vi "replaceGoto.vi"(10 "String in":string) -> (2 "BotSpeak Out":string)   [LabVIEW 2012]
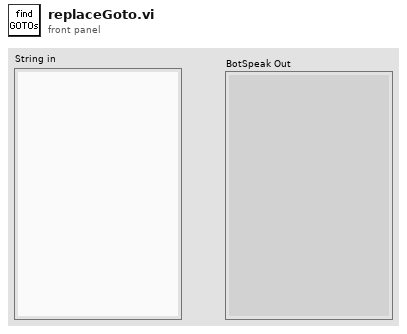
[diagram p1: front panel]
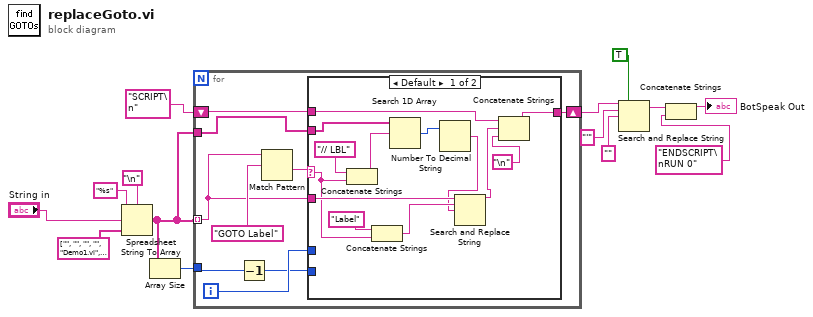
[diagram p0: block diagram]
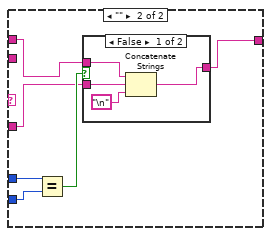
[diagram p2: hidden frame]
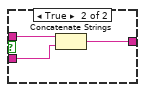
[diagram p3: hidden frame]
diagram:
  n1 = Spreadsheet String To Array(delimiter (Tab)="\n", format string="%s", spreadsheet string="String in", array type (2D Dbl)=string[] ["", "", "", "", "Demo1.vi", "DigitalWrite.vi", "VS_Wait.vi", ""] ("Array 3")) -> (array=w7:string[])
  n2 = Array Size(array=w7) -> (size(s)=w6:i32)
  n3 = for {
    tunnel: w7 -> [w20] mode=indexing
    tunnel: w7 -> [w23]
    shift-right: [w15] -> w2
    shift-left: "SCRIPT\n" -> [w22]
    tunnel: w6 -> [w16]
    i -> [w18]
    n4 = Decrement(x=w16) -> (x-1=w17:i32)
    n5 = Match Pattern(string=w20, regular expression="GOTO Label" ("search string/char (-)")) -> (after substring=w19:string)  [unwired: 1 in, 3 out]
    n6 = case shown="Default" w19 {
      selector: w19 -> [w32 _]
      tunnel: w23 -> [w36 _]
      tunnel: w20 -> [w33 w38]
      tunnel: [w25 w37] -> w15
      tunnel: w22 -> [w27 w39]
      tunnel: w18 -> [_ w42]
      tunnel: w17 -> [_ w41]
      frame Default {
        n7 = Concatenate Strings("// LBL" ("string"), w32) -> (w34:string)
        n8 = Concatenate Strings("Label" ("string"), w32) -> (w30:string)
        n9 = Search 1D Array(1D array=w36, element=w34) -> (index of element=w29:i32)  [unwired: 1 in]
        n10 = Number To Decimal String(number=w29) -> (decimal integer string=w28:string)  [unwired: 1 in]
        n11 = Search and Replace String(input string=w33, search string=w30, replace string=w28) -> (result string=w26:string)  [unwired: 5 in, 3 out]
        n12 = Concatenate Strings(w27, w26, "\n") -> (w25:string)
      }
      frame "" {
        n13 = Equal?(x=w42, y=w41) -> (x = y?=w40:bool)
        n14 = case shown="False" w40 {
          tunnel: w39 -> [w46 w49]
          tunnel: w38 -> [w45 w48]
          tunnel: [w43 w47] -> w37
          frame False {
            n15 = Concatenate Strings(w46, w45, "\n") -> (w43:string)
          }
          frame True {
            n16 = Concatenate Strings(w49, w48) -> (w47:string)
          }
        }
      }
    }
  }
  n17 = Search and Replace String(replace all?=TRUE ("replace all? (F)"), input string=w2, search string="'", replace string="" ("replace string (\"\")")) -> (result string=w1:string)  [unwired: 4 in, 3 out]
  n18 = Concatenate Strings(w1, "ENDSCRIPT\nRUN 0" ("string")) -> (→"BotSpeak Out":string)
